vi "SetParam.vi"(8 "error in (no error)":errorcluster caption="entrée d'erreur (pas d'erreur)", 10 "pairwise_kernels":T1={"metric "="linear", "filter_params"=FALSE, "n_jobs"="None"}, 11 "Pairwise_kernels.lvclass":refnum<class "Pairwise_kernels.lvclass">) -> (0 "error out":errorcluster caption="sortie d'erreur", 3 "Pairwise_kernels.lvclass":refnum<class "Pairwise_kernels.lvclass">)   [LabVIEW 2020, in "Pairwise_kernels.lvclass"]
doc: "Set Parameters"
uses:
  Pairwise_kernels.lvclass
  Pairwise_kernels.lvclass/Pairwise_kernels.ctl
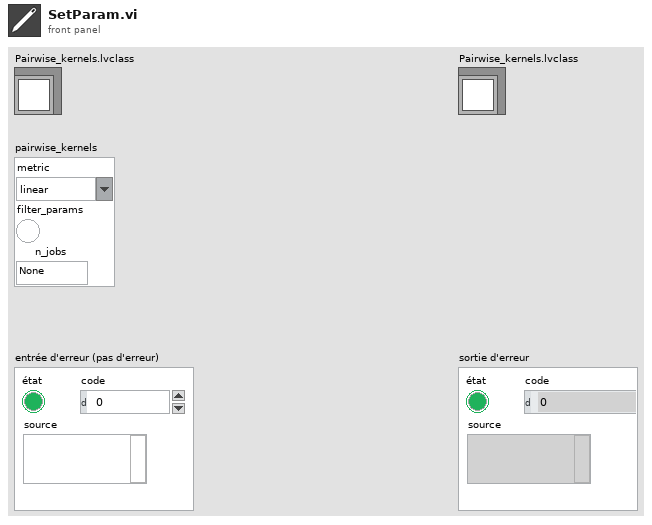
[diagram p1: front panel]
types:
  T1 = cluster{"metric ":string, "filter_params":bool, "n_jobs":string}
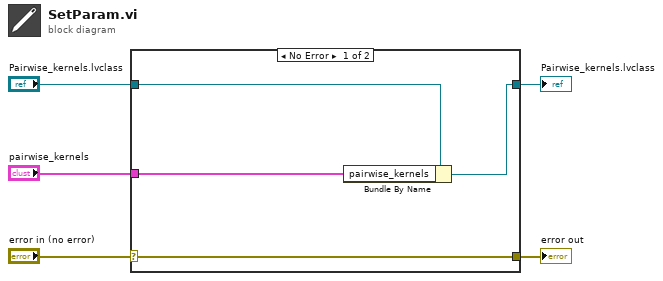
[diagram p0: block diagram]
diagram:
  n1 = case shown="No Error" "error in (no error)" {
    selector: "error in (no error)" -> [w9 w10]
    tunnel: [w9 w10] -> w4
    tunnel: [w7 w11] -> w2
    tunnel: "Pairwise_kernels.lvclass" -> [w8 w11]
    tunnel: "pairwise_kernels" -> [w6 _]
    frame No Error {
      n2 = Bundle By Name(cluster=w8, "pairwise_kernels"=w6) -> (w7:refnum<class "Pairwise_kernels.lvclass">)
    }
    frame Error {
    }
  }
  "error out" <- w4
  "Pairwise_kernels.lvclass" <- w2
